vi "Data Conversion.vi"() -> ()   [LabVIEW 2013]
uses:
  <vilib>/Utility/file.llb/Write To Spreadsheet File (DBL).vi
panel:
  in  "Tab Control":enum32{"File and Quick View", "Detailed View"}(tab)
  in  "File name for file to open: (set .tdms file extension)":string="EW_TC_Run_2.tdms"
  in  "Path for file to open":string="C:\\Users\\Public\\Documents\\Dual Crank Engine\\Test Rig Results\\Ed Winward\\2015-01-08\\Saved to Chassis"
  out "CSV file saved as:":path
  in  "File name for the file to save: (set .csv file extension)":string="EW_TC_Run_2.csv"
  in  "Save to a CSV File?":bool
  in  "Path for the file to save":string="C:\\Users\\Public\\Documents\\Dual Crank Engine\\Test Rig Results\\Ed Winward\\2015-01-08\\Saved to Chassis"
  out "CSV Output file generated?":bool
  out "Sample Time, sec":dbl[](array[numeric])
  out "Crank Position, rev":dbl[](array[numeric])
  out "Crank Speed, rev/s":dbl[](array[numeric])
  out "Motor Torque, Nm":dbl[](array[numeric])
  out "Load Cell Force, N":dbl[](array[numeric])
  out "Data Display":dbl[][](graph)
  out "Data Display 2":dbl[][](graph)
  # "Twin Crank Rig TDMS Data File Plotter and Converter"
  # "File To Open:"
  # "Raw Data Plot"
  # "Use Windows explorer to find the directory and then\ncopy paste this directory into the above box"
  # "Use Windows explorer to find the directory and then\ncopy paste this directory into the above box"
  # "Use the magnifying icon to zoom around the plot"
  # "Raw Data Plot"
  # "Use the magnifying icon to zoom around the plot"
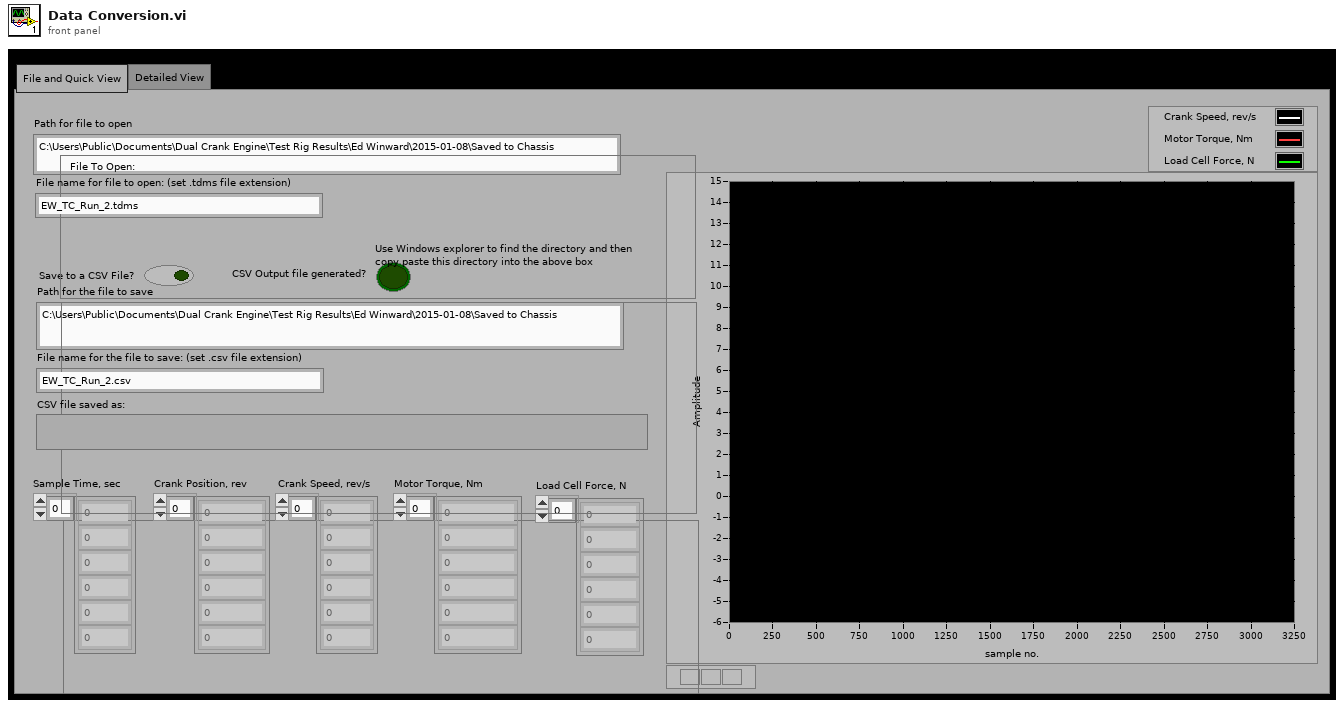
[diagram p1: front panel]
types:
  T1 = enum16{"big-endian, network order", "native, host order", "little-endian"}
  T2 = enum16{"open", "open or create", "create or replace", "create", "open (read-only)"}
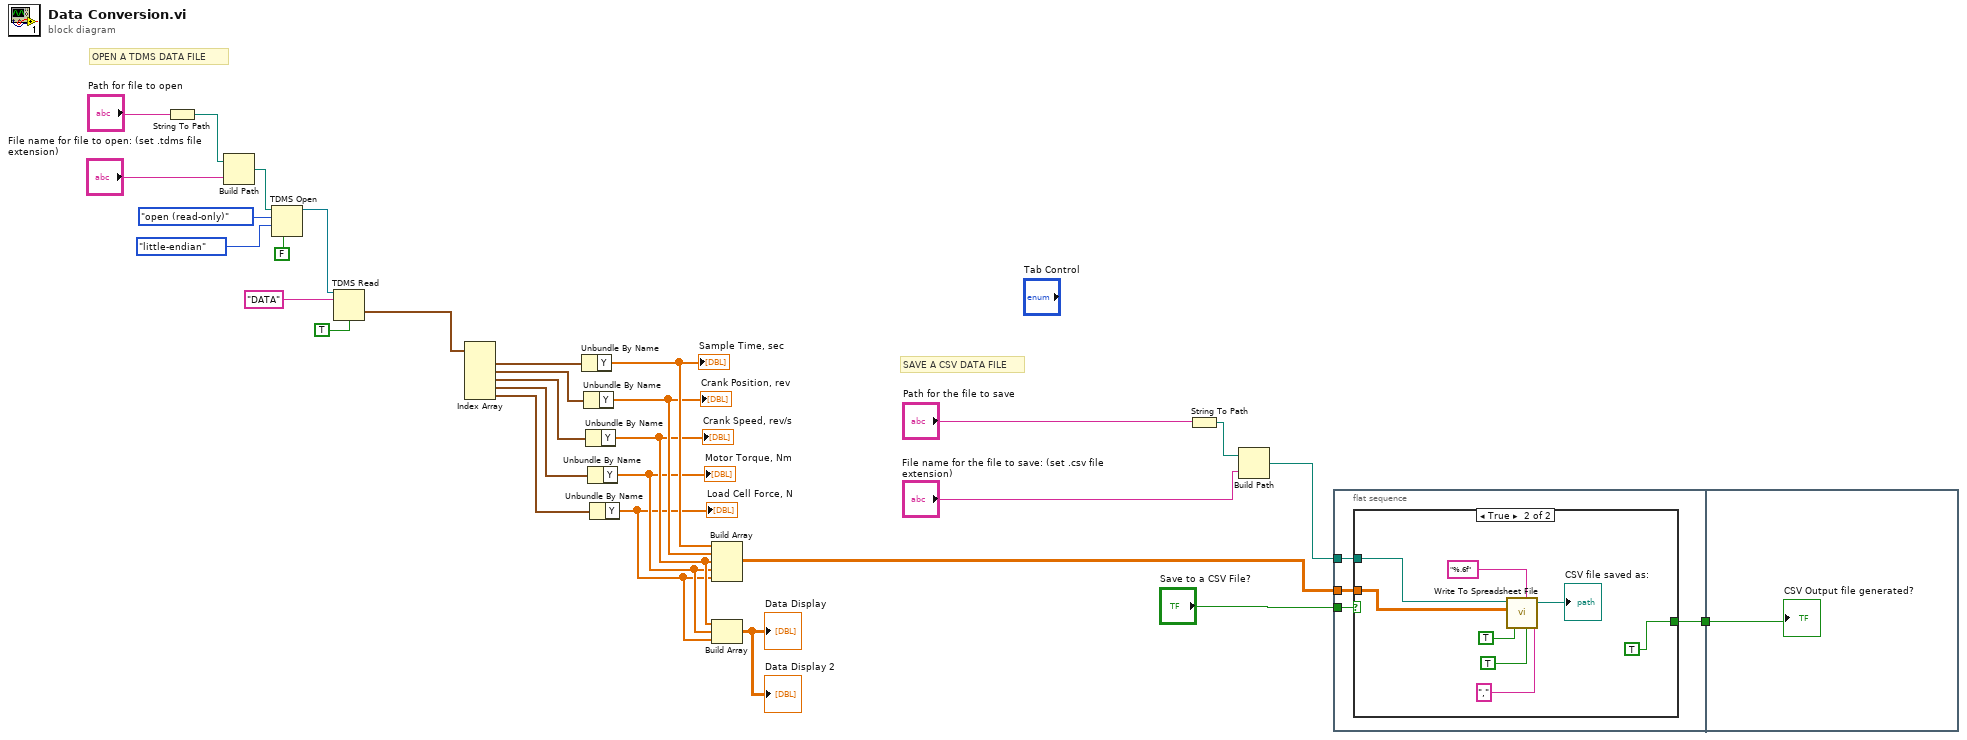
[diagram p0: block diagram]
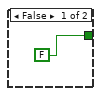
[diagram p2: hidden frame]
diagram:
  # "OPEN A TDMS DATA FILE"
  # "SAVE A CSV DATA FILE"
  n1 = String To Path(string="Path for file to open") -> (path=w5:path)
  n2 = Build Path(base path=w5, name or relative path="File name for file to open: (set .tdms file extension)") -> (appended path=w25:path)
  n3 = TDMS Open(6:FALSE ("disable buffering (T)"), 9:T1."little-endian" ("byte order (2:little-endian)"), 10:T2."open (read-only)" ("operation"), 11:w25) -> (3:w26:refnum<k34>)  [unwired: 3 in, 1 out]
  n4 = TDMS Read(0:w26, 5:"DATA" ("group name in (Untitled)"), 13:TRUE ("return channels in file order? (F)")) -> (10:w21:waveform(dbl)[])  [unwired: 5 in, 5 out]
  n5 = Index Array(array=w21) -> (element #1=w20:waveform(dbl), element #2=w19:waveform(dbl), element #3=w18:waveform(dbl), element #4=w17:waveform(dbl), element #5=w16:waveform(dbl))  [unwired: 5 in]
  n6 = Unbundle By Name(w20) -> ("Y"=w12:dbl[])
  "Sample Time, sec" <- w12
  n7 = Unbundle By Name(w19) -> ("Y"=w10:dbl[])
  "Crank Position, rev" <- w10
  n8 = Unbundle By Name(w18) -> ("Y"=w9:dbl[])
  "Crank Speed, rev/s" <- w9
  n9 = Unbundle By Name(w17) -> ("Y"=w8:dbl[])
  "Motor Torque, Nm" <- w8
  n10 = Unbundle By Name(w16) -> ("Y"=w7:dbl[])
  "Load Cell Force, N" <- w7
  n11 = Build Array(w12, w10, w9, w8, w7) -> (w11:dbl[][])
  n12 = Build Array(w9, w8, w7) -> (→"Data Display" →"Data Display 2":dbl[][])
  n13 = String To Path(string="Path for the file to save") -> (path=w3:path)
  n14 = Build Path(base path=w3, name or relative path="File name for the file to save: (set .csv file extension)") -> (appended path=w13:path)
  n15 = flat-sequence {
    tunnel: "Save to a CSV File?" -> [w33]
    tunnel: w13 -> [w32]
    tunnel: w11 -> [w31]
    tunnel: [w30] -> w2
    tunnel: w2 -> [w43]
    frame #0 {
      n16 = case shown="True" w33 {
        tunnel: w32 -> [_ w38]
        tunnel: w31 -> [_ w37]
        tunnel: [FALSE TRUE] -> w30
        frame False {
        }
        frame True {
          n17 = call-poly <vilib>:"Write To Spreadsheet File.vi"("delimiter (\\t)"="," ("delimiter (\\t)"), "transpose? (no:F)"=TRUE, "format (%.3f)"="%.6f", "append to file? (new file:F)"=TRUE, "2D data"=w37, "file path (dialog if empty)"=w38) -> ("new file path (Not A Path if cancelled)"=→"CSV file saved as:":path)  [unwired: 2 in]
        }
      }
    }
    frame #1 {
      "CSV Output file generated?" <- w43
    }
  }
